vi "ObjectEditorLauncher.vi"   [LabVIEW 2022 SP3]
uses:
  Components/ViPER.lvlibp/ViPER.lvclass
panel:
  # "OBJECT EDITOR"
types:
  T1 = enum32{"Invalid", "Standard", "Closed", "Hidden", "Minimized", "Maximized"}
  T2 = enum32{"invalid app kind", "Development System", "Run Time System", "Student Edition", "Embedded LabVIEW", "Evaluation", "Custom"}
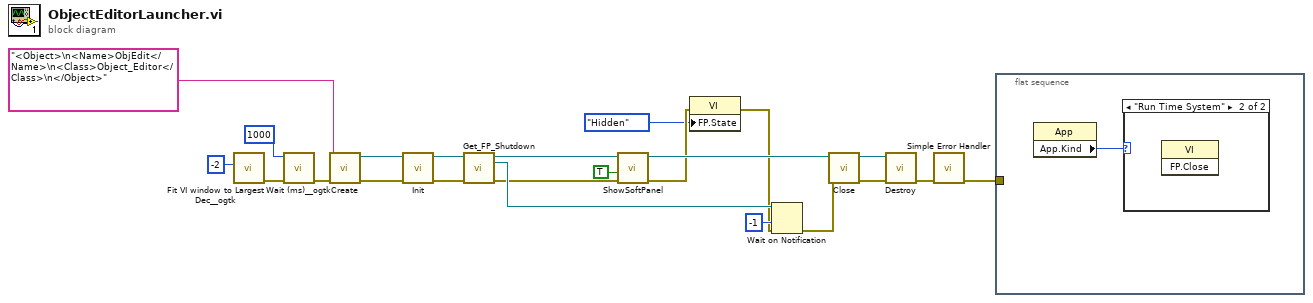
[diagram p0: block diagram]
diagram:
  n1 = call <userlib>:"Fit VI window to Largest Dec__ogtk.vi"("border spacing (2 px)"=-2) -> ("error out"=w3:errorcluster)  [unwired: 5 in, 1 out]
  n2 = call <userlib>:"Wait (ms)__ogtk.vi"("error in (no error)"=w3, "milliseconds to wait"=u32 1000) -> ("error out"=w2:errorcluster)  [unwired: 8 in, 1 out]
  n3 = call "Create.vi"("error in (no error)"=w2, "Config XML"="<Object>\n<Name>ObjEdit</Name>\n<Class>Object_Editor</Class>\n</Object>") -> ("error out"=w19:errorcluster, "reference out"=w20:refnum<class "ViPER.lvclass">)  [unwired: 8 in]
  n4 = call-dynamic "Init.vi"("error in (no error)"=w19, "reference in"=w20) -> ("error out"=w17:errorcluster, "reference out"=w18:refnum<class "ViPER.lvclass">)  [unwired: 8 in]
  n5 = call "Get_FP_Shutdown.vi"("ViPER_Base in"=w18, "error in (no error)"=w17) -> ("ViPER_Base out"=w15:refnum<class "ViPER.lvclass">, "SoftFP_Shutdown"=w16:refnum<notifier>, "error out"=w14:errorcluster)  [unwired: 10 in, 1 out]
  n6 = call-dynamic "ShowSoftPanel.vi"("error in (no error)"=w14, "Floating"=TRUE, "Driver in"=w15) -> ("error out"=w6:errorcluster, "Driver out"=w13:refnum<class "ViPER.lvclass">)  [unwired: 6 in, 1 out]
  n7 = property class="VI"(error in=w6, "FP.State"=T1."Hidden" ("Front Panel Window:State")) -> (error out=w5:errorcluster)  [unwired: 1 in, 1 out]
  n8 = Wait on Notification(notifier=w16, timeout in ms (-1)=-1, error in (no error)=w5) -> (error out=w23:errorcluster)  [unwired: 1 in, 3 out]
  n9 = call-dynamic "Close.vi"("error in (no error)"=w23, "reference in"=w13) -> ("error out"=w12:errorcluster, "reference out"=w10:refnum<class "ViPER.lvclass">)  [unwired: 8 in]
  n10 = call "Destroy.vi"("error in (no error)"=w12, "reference in"=w10) -> ("error out"=w11:errorcluster)  [unwired: 9 in]
  n11 = call <vilib>:"Simple Error Handler.vi"("error in (no error)"=w11) -> ("error out"=w8:errorcluster)  [unwired: 4 in, 4 out]
  n12 = flat-sequence {
    tunnel: w8 -> [_]
    frame #0 {
      n13 = property class="App"() -> ("App.Kind"=w24:T2)  [unwired: 2 in, 2 out]
      n14 = case shown="\"Run Time System\"" w24 {
        frame "invalid app kind", Default {
        }
        frame "Run Time System" {
          n15 = invoke class="VI" method="FP.Close"() -> ()  [unwired: 3 in, 3 out]
        }
      }
    }
  }
